vi "Localisation.vi"() -> ()   [LabVIEW 2009]
uses:
  user32.dll
panel:
  in  "EARTHLib.IApplicationGE":refnum<k7>
  in  "WebBrowser":refnum<k7>(container)
  out "hWnd 3":u32
  out "hWnd 2":u32
  out "hWnd":u32
  out "GetRenderHwnd":i32
  out "AutoPilotSpeed":dbl
  out "StreamingProgressPercentage":i32(slide) scale=0.0..100.0
  in  "stop":bool
  in  "Set View Position":T1={"Azimuth"=0.0, "Latitude"=51.4061, "Longitude"=-1.30684, "Range"=50000.0, "Tilt"=0.0} {"Azimuth" min=-180.0 max=180.0; "Latitude" min=-180.0 max=180.0; "Longitude" min=-180.0 max=180.0; "Range" min=0.0; "Tilt" min=0.0 max=90.0}
  in  "terrain":i32 min=0 max=1
  in  "Set":bool
  out "data":dbl[](array[numeric])
  in  "screen_x":dbl min=0.0
  in  "screen_y":dbl min=0.0
  out "View Position":T2
  out "VersionAppType":i32(ring)=255 items=["EnterpriseClientGE"=0, "ProGE"=1, "PlusGE"=2, "FreeGE"=5, "UnknownGE"=255]
  out "VersionMajor":i32
  out "VersionMinor":i32
  out "VersionBuild":i32
  in  "KML Path":path
  in  "error in":errorcluster
  in  "EARTHLib.IKHInterface":refnum<k7>
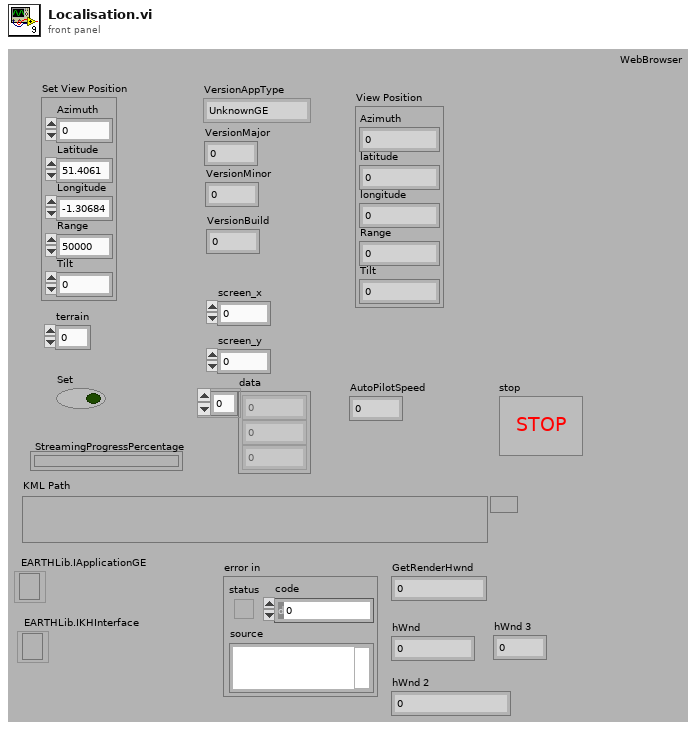
[diagram p1: front panel]
types:
  T1 = cluster{"Azimuth":dbl, "Latitude":dbl, "Longitude":dbl, "Range":dbl, "Tilt":dbl}
  T2 = cluster{"Azimuth":dbl, "latitude":dbl, "longitude":dbl, "Range":dbl, "Tilt":dbl}
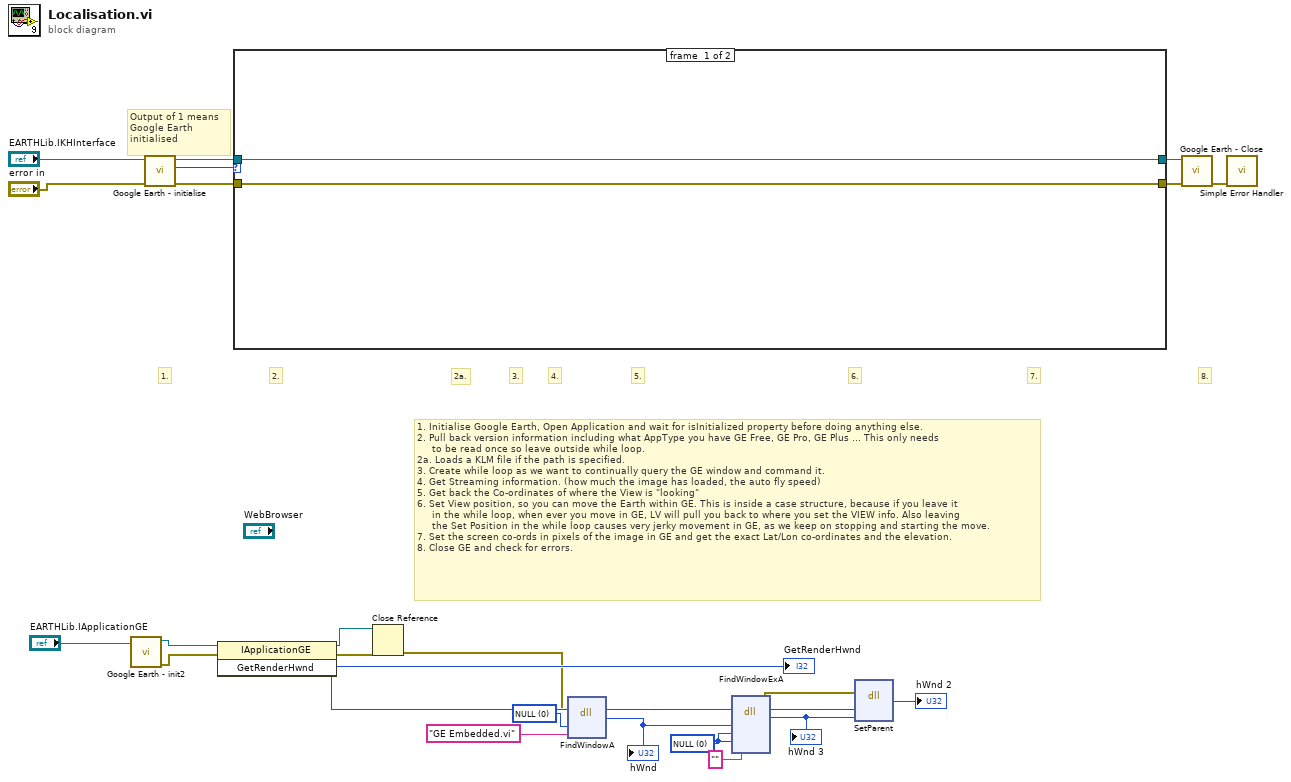
[diagram p0: block diagram]
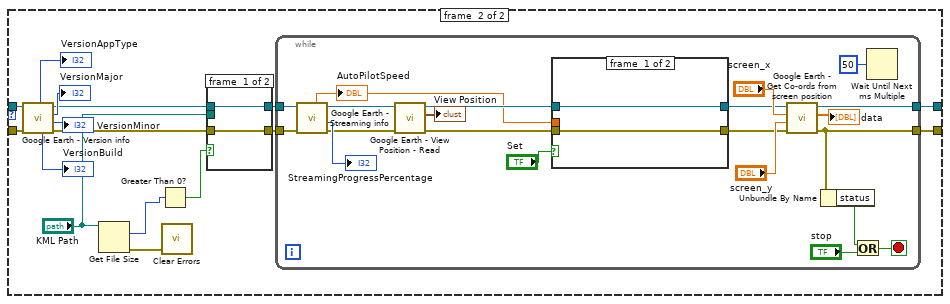
[diagram p2: hidden frame]
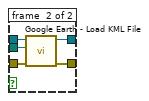
[diagram p3: hidden frame]
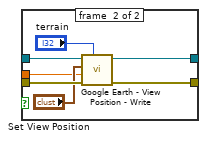
[diagram p4: hidden frame]
diagram:
  w11 = 0 items=["NULL"]
  w15 = 0 items=["NULL"]
  # "2a."
  # "1. Initialise Google Earth, Open Application and wait for isInitialized property before doing anything else.\n2. Pull back version information including what AppType you have GE Free, GE Pro, GE Plus ... This only needs\n     to be read once so leave outside while loop.\n2a. Loads a KLM file if the path is specified.\n3. Create while loop as we want to continually query the GE window and command it.\n4. Get Streaming information. (how much the image has loaded, the auto fly speed)\n5. Get back the Co-ordinates of where the View is \"looking\"\n6. Set View position, so you can move the Earth within GE. This is inside a case structure, because if you leave it \n     in the while loop, when ever you move in GE, LV will pull you back to where you set the VIEW info. Also leaving\n     the Set Position in the while loop causes very jerky movement in GE, as we keep on stopping and starting the move.\n7. Set the screen co-ords in pixels of the image in GE and get the exact Lat/Lon co-ordinates and the elevation.\n8. Close GE and check for errors."
  # "8."
  # "7."
  # "6."
  # "5."
  # "4."
  # "3."
  # "2."
  # "1."
  # "Output of 1 means\nGoogle Earth \ninitialised"
  n1 = call "Google Earth - init2.vi"("EARTHLib.IApplicationGE"="EARTHLib.IApplicationGE") -> ("error out"=w1:errorcluster, "Refnum Out"=w2:refnum<k7>)  [unwired: 8 in, 1 out]
  n2 = call "Google Earth - initialise.vi"("error in (no error)"="error in", "EARTHLib.IKHInterface"="EARTHLib.IKHInterface") -> ("error out"=w4:errorcluster, "IsInitialized"=w23:i32, "Refnum Out"=w5:refnum<k7>)  [unwired: 7 in]
  n3 = invoke class="IApplicationGE" method="GetRenderHwnd"(reference=w2, error in=w1) -> (reference out=w17:refnum<k7>, error out=w18:errorcluster, "GetRenderHwnd"=w14:i32)  [unwired: 1 in]
  "GetRenderHwnd" <- w14
  n4 = case shown="1" w23 {
    tunnel: w5 -> [w25 w40]
    tunnel: w4 -> [w26 w41]
    tunnel: [w26 w42] -> w21
    tunnel: [w25 w35] -> w20
    frame #0 {
    }
    frame #1 {
      n5 = call "Google Earth - Version info.vi"("error in"=w41, "Refnum In"=w40) -> ("error out"=w32:errorcluster, "VersionMinor"=→"VersionMinor":i32, "VersionMajor"=→"VersionMajor":i32, "Refnum Out"=w34:refnum<k7>, "VersionBuild"=→"VersionBuild":i32, "VersionAppType"=→"VersionAppType":i32)  [unwired: 4 in]
      n6 = Get File Size(file="KML Path") -> (size (in bytes)=w29:i64, 0:w28:errorcluster)  [unwired: 1 in, 1 out]
      n7 = Greater Than 0?(x=w29) -> (x > 0?=w30:bool)
      n8 = call <vilib>:"Clear Errors.vi"("error in (no error)"=w28) -> ()  [unwired: 6 in, 1 out]
      n9 = case shown="True" w30 {
        tunnel: w34 -> [w44 w49]
        tunnel: [w44 w48] -> w33
        tunnel: w32 -> [w43 w47]
        tunnel: [w43 w46] -> w31
        tunnel: "KML Path" -> [_ w45]
        frame #0 {
        }
        frame #1 {
          n10 = call "Google Earth - Load KML File.vi"("error in"=w47, "KML Path"=w45, "Refnum in"=w49) -> ("error out"=w46:errorcluster, "Refnum Out"=w48:refnum<k7>)  [unwired: 7 in]
        }
      }
      n11 = while {
        tunnel: w33 -> [w57]
        tunnel: w31 -> [w70]
        tunnel: [w53] -> w42
        tunnel: [w54] -> w35
        stop <- w50 stop-if-true
        n12 = call "Google Earth - Streaming info.vi"("error in"=w70, "Refnum in"=w57) -> ("error out"=w68:errorcluster, "StreamingProgressPercentage"=→"StreamingProgressPercentage":i32, "Refnum Out"=w56:refnum<k7>, "AutoPilotSpeed"=w65:dbl)  [unwired: 6 in]
        "AutoPilotSpeed" <- w65
        n13 = call "Google Earth - View Position - Read.vi"("error in"=w68, "Refnum in"=w56) -> ("error out"=w66:errorcluster, "Camera Position"=→"View Position":T2, "Refnum Out"=w67:refnum<k7>)  [unwired: 7 in]
        n14 = case shown="True" "Set" {
          tunnel: w67 -> [w71 w79]
          tunnel: w66 -> [w72 w78]
          tunnel: [w72 w77] -> w60
          tunnel: w65 -> [_ w75]
          tunnel: [w71 w74] -> w59
          frame #0 {
          }
          frame #1 {
            n15 = call "Google Earth - View Position - Write.vi"("terrain"="terrain", "error in"=w78, "speed"=w75, "Camera Position"="Set View Position", "Refnum in"=w79) -> ("error out"=w77:errorcluster, "Refnum Out"=w74:refnum<k7>)  [unwired: 5 in]
          }
        }
        n16 = call "Google Earth - Get Co-ords from screen position.vi"("error in"=w60, "screen_y"="screen_y", "screen_x"="screen_x", "Refnum In"=w59) -> ("error out"=w53:errorcluster, "data"=→"data":dbl[], "RefnumOut"=w54:refnum<k7>)  [unwired: 5 in]
        n17 = Unbundle By Name(w53) -> ("status"=w52:bool)
        n18 = Or(x=w52, y="stop") -> (x .or. y?=w50:bool)
        n19 = Wait Until Next ms Multiple(millisecond multiple=u32 50 ("milliseconds to wait")) -> ()  [unwired: 1 out]
      }
    }
  }
  n20 = Close Reference(reference=w17, error in (no error)=w18) -> (error out=w13:errorcluster)
  n21 = dll-call lib="user32.dll" fn="FindWindowA" label="FindWindow"(error in=w13, "lpszClassName"=w15, "lpszWindowName"="GE Embedded.vi" ("window name (\"\")")) -> (error out=w8:errorcluster, "hWnd"=w12:u32)  [unwired: 3 in, 2 out]
  "hWnd" <- w12
  n22 = dll-call lib="user32.dll" fn="FindWindowExA" label="Find Child"(error in=w8, "Parent HWND"=w12, "Child_After HWND"=w11, "lpszClassName"=w11, "lpszWindowName"="") -> (error out=w7:errorcluster, "hWnd"=w10:u32)  [unwired: 5 in, 2 out]
  "hWnd 3" <- w10
  n23 = dll-call lib="user32.dll" fn="SetParent" label="Set Parent"(error in=w7, "hWndChild"=w14, "hWndNewParent"=w10) -> ("hWnd"=→"hWnd 2":u32)  [unwired: 4 in, 2 out]
  n24 = call "Google Earth - Close.vi"("error out"=w21, "Refnum In"=w20) -> ("error out 2"=w19:errorcluster)  [unwired: 9 in]
  n25 = call <vilib>:"Simple Error Handler.vi"("error in (no error)"=w19) -> ()  [unwired: 4 in, 5 out]
